vi "NavbalLabVIEW(15-5-21).vi"() -> ()   [LabVIEW 2010] (continued)
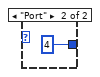
[diagram p2: hidden frame]
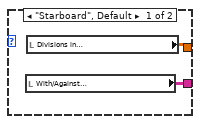
[diagram p4: hidden frame]
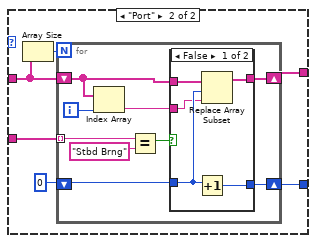
[diagram p6: hidden frame]
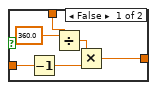
[diagram p10: hidden frame]
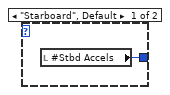
[diagram p11: hidden frame]
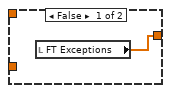
[diagram p12: hidden frame]
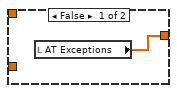
[diagram p13: hidden frame]
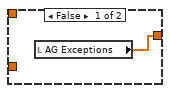
[diagram p14: hidden frame]
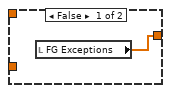
[diagram p15: hidden frame]
                  n2665 = Decrement(x=w3078) -> (x-1=w3116:dbl)
                  n2666 = Decrement(x=w3079) -> (x-1=w3115:dbl)
                  n2667 = Decrement(x=w3077) -> (x-1=w3117:dbl)
                  n2668 = Multiply(x=w3116, y=w3068) -> (x*y=w3090:dbl)
                  n2669 = Multiply(x=w3115, y=w3068) -> (x*y=w3080:dbl)
                  n2670 = Multiply(x=w3117, y=w3068) -> (x*y=w3109:dbl)
                  n2671 = Build Array (concatenate) "Percent"(w3137, w3138) -> (w3133:T3)
                  n2672 = Index Array(array=w3111, index (row)=w3080, index (col)=w3081) -> (element=w3112:bool)
                  n2673 = Index Array(array=w3111, index (row)=w3090, index (col)=w3091) -> (element=w3113:bool)
                  n2674 = Index Array(array=w3111, index (row)=w3109, index (col)=w3108) -> (element=w3114:bool)
                  n2675 = Index Array(array=w3076, index (row)=w3090, index (col)=w3091) -> (element=w3092:dbl)
                  n2676 = Index Array(array=w3076, index (row)=w3109, index (col)=w3108) -> (element=w3105:dbl)
                  n2677 = Index Array(array=w3076, index (row)=w3080, index (col)=w3081) -> (element=w3087:dbl)
                  n2678 = Greater Than 0?(x=w3092) -> (x > 0?=w3089:bool)
                  n2679 = Greater Than 0?(x=w3105) -> (x > 0?=w3106:bool)
                  n2680 = Greater Than 0?(x=w3087) -> (x > 0?=w3083:bool)
                  n2681 = Number To Fractional String(number=w3092, precision (6)=i16 1) -> (F-format string=w3093:string)  [unwired: 2 in]
                  n2682 = Number To Fractional String(number=w3105, precision (6)=i16 1) -> (F-format string=w3104:string)  [unwired: 2 in]
                  n2683 = Number To Fractional String(number=w3087, precision (6)=i16 1) -> (F-format string=w3086:string)  [unwired: 2 in]
                  n2684 = Concatenate Strings(w3093, " wt in hole") -> (w3088:string)
                  n2685 = Concatenate Strings(w3104, " wt in hole") -> (w3102:string)
                  n2686 = Concatenate Strings(w3086, " wt in hole") -> (w3082:string)
                  n2687 = Build Array (concatenate)(w3135, w3133) -> (w3134:T3)
                  n2688 = Select(t=w3082, s=w3083, f="  ") -> (s? t:f=w3096:string)
                  n2689 = Select(t=w3102, s=w3106, f="  ") -> (s? t:f=w3100:string)
                  n2690 = Select(t=w3088, s=w3089, f="  ") -> (s? t:f=w3098:string)
                  n2691 = Number To Fractional String(number=w3134, precision (6)=i16 3) -> (F-format string=w3132:string[][])  [unwired: 2 in]
                  n2692 = Build Array(w3129, w3129, w3129, w3129) -> (w3131:string[])
                  n2693 = Select(t=w3121, s=w3112, f=w3096) -> (s? t:f=w3124:string)
                  n2694 = Select(t=w3121, s=w3113, f=w3098) -> (s? t:f=w3123:string)
                  n2695 = Select(t=w3121, s=w3114, f=w3100) -> (s? t:f=w3122:string)
                  n2696 = Insert Into Array(array=w3132, index (row)=1, new element=w3131) -> (w3128:string[][])  [unwired: 1 in]
                  n2697 = Replace Array Subset(array=w3128, new element=w3129, index (row)=3 ("disabled index (row)"), index (col)=0 ("disabled index (col)")) -> (w3119:string[][])
                  n2698 = Build Array(w3124, "  ", w3123, w3122) -> (w3120:string[])
                  n2699 = Insert Into Array(array=w3119, index (col)=4 ("disabled index (col)"), new element=w3120) -> (w3118:string[][])  [unwired: 1 in]
                  n2700 = property on="Fwd Generator Balance Plane Split Options" class="MCListbox (strict)"("ItemNames"=w3118) -> ()  [unwired: 2 in, 2 out]
                  "FG Correction 1" <- w3069
                  "FG Correction 2A" <- w3072
                  "FG Correction 2B" <- w3071
                }
              }
            }
            "2wt-Exceptions" <- w2654
          }
        }
        n2701 = local read "AT Exceptions"() -> (w621:csg[])
        n2702 = local read "2wt-Exceptions"() -> (w620:csg[])
        n2703 = case shown="True" "Omit AT" {
          tunnel: w621 -> [_ w839]
          tunnel: w620 -> [_ w837]
          tunnel: [w833 w834] -> w619
          frame False {
            n2704 = local read "AT Exceptions"() -> (w833:csg[])
          }
          frame True {
            n2705 = Index Array(array=w837, index=0) -> (element=w835:csg)
            n2706 = Insert Into Array(array=w839, index=0, new element=w835) -> (w834:csg[])
          }
        }
        "AT Exceptions" <- w619
        n2707 = local read "FT Exceptions"() -> (w615:csg[])
        n2708 = local read "2wt-Exceptions"() -> (w616:csg[])
        n2709 = case shown="True" "Omit FT" {
          tunnel: w615 -> [_ w832]
          tunnel: w616 -> [_ w830]
          tunnel: [w826 w827] -> w617
          frame False {
            n2710 = local read "FT Exceptions"() -> (w826:csg[])
          }
          frame True {
            n2711 = Index Array(array=w830, index=1) -> (element=w828:csg)
            n2712 = Insert Into Array(array=w832, index=0, new element=w828) -> (w827:csg[])
          }
        }
        "FT Exceptions" <- w617
        n2713 = local read "AG Exceptions"() -> (w623:csg[])
        n2714 = local read "2wt-Exceptions"() -> (w624:csg[])
        n2715 = case shown="True" "Omit AG" {
          tunnel: w623 -> [_ w846]
          tunnel: w624 -> [_ w844]
          tunnel: [w840 w841] -> w625
          frame False {
            n2716 = local read "AG Exceptions"() -> (w840:csg[])
          }
          frame True {
            n2717 = Index Array(array=w844, index=2) -> (element=w842:csg)
            n2718 = Insert Into Array(array=w846, index=0, new element=w842) -> (w841:csg[])
          }
        }
        "AG Exceptions" <- w625
        n2719 = local read "FG Exceptions"() -> (w628:csg[])
        n2720 = local read "2wt-Exceptions"() -> (w627:csg[])
        n2721 = case shown="True" "Omit FG" {
          tunnel: w628 -> [_ w853]
          tunnel: w627 -> [_ w851]
          tunnel: [w847 w848] -> w626
          frame False {
            n2722 = local read "FG Exceptions"() -> (w847:csg[])
          }
          frame True {
            n2723 = Index Array(array=w851, index=3) -> (element=w849:csg)
            n2724 = Insert Into Array(array=w853, index=0, new element=w849) -> (w848:csg[])
          }
        }
        "FG Exceptions" <- w626
        n2725 = local read "Divisions in\nEach Plane"() -> (w636:T3)
        n2726 = local read "1st Available"() -> (w650:bool)
        n2727 = local read "2nd Available"() -> (w649:bool)
        n2728 = local read "3rd Available"() -> (w648:bool)
        n2729 = local read "4th Available"() -> (w647:bool)
        n2730 = case shown="True" w650 {
          tunnel: w636 -> [_ w1024]
          frame False {
          }
          frame True {
            n2731 = invoke on="Aft Turbine Balance Plane Split Options" class="MCListbox (strict)" method="Get DblClk Row"() -> ("Get Double-clicked Row"=w1025:i32)  [unwired: 3 in, 2 out]
            n2732 = Index Array(array=w1024, index (row)=0, index (col)=0 ("disabled index (col)")) -> (element=w1022:dbl)
            n2733 = case shown="2" w1025 {
              tunnel: w1022 -> [_ w1026 w1053]
              frame -2, Default {
                # "-2 is the variable value when no box is currently double clicked"
              }
              frame 0 {
                w1030 = 360.0 ("x")
                w1042 = 0 ("disabled index (col)")
                w1046 = 0 ("disabled index (col)")
                # "Update Pending weights Boolean Array\nwith selected split's locations"
                # "Update Inputs for Prediction tab\nto reflect selected weight split"
                # "Pull mass, Phase, and Location Data\nfrom listbox's array"
                # "Single Mass Option Selected"
                n2734 = local read "AT Correction 1"() -> (w1040:cdb)
                n2735 = Complex To Polar(r * e^(i*theta)=w1040) -> (r=w1039:dbl, theta=w1027:dbl)
                n2736 = Divide(x=w1027, y=3.141592653589793) -> (x/y=w1038:dbl)
                n2737 = local read "Correction Mag"() -> (w1047:T3)
                n2738 = Multiply ("Multiply.vi")(x=180.0, y=w1038) -> (x*y=w1033:dbl)
                n2739 = Add ("Add.vi")(x=w1033, y=w1030) -> (x+y=w1034:dbl)
                n2740 = Greater Than 0?(x=w1033) -> (x > 0?=w1035:bool)
                n2741 = Select(t=w1033, s=w1035, f=w1034) -> (s? t:f=w1032:dbl)
                n2742 = Divide(x=w1026, y=w1030) -> (x/y=w1031:dbl)
                n2743 = Replace Array Subset(array=w1047, new element=w1039, index (row)=w1046, index (col)=w1046) -> (w1045:T3)
                n2744 = Multiply ("Multiply.vi")(x=w1032, y=w1031) -> (x*y=w1029:dbl)
                n2745 = Increment(x=w1029) -> (x+1=w1028:dbl)
                n2746 = local read "Correction Loc"() -> (w1044:T3)
                n2747 = local write "Correction Mag"(w1045) -> ()
                n2748 = Replace Array Subset(array=w1044, new element=w1028, index (row)=w1042, index (col)=w1042) -> (w1043:T3)
                n2749 = local write "Correction Loc"(w1043) -> ()
                n2750 = property on="Aft Turbine Balance Plane Split Options" class="MCListbox (strict)"("SelColor"=u32 40727) -> ()  [unwired: 2 in, 2 out]
              }
              frame 2 {
                w1052 = 360.0 ("x")
                w1066 = 0 ("disabled index (col)")
                w1070 = 0 ("disabled index (col)")
                n2751 = local read "AT Correction 2A"() -> (w1048:cdb)
                n2752 = local read "AT Correction 2B"() -> (w1049:cdb)
                n2753 = local read "Correction Mag"() -> (w1071:T3)
                n2754 = Add ("Add.vi")(x=w1048, y=w1049) -> (x+y=w1065:cdb)
                n2755 = Complex To Polar ("Complex To Polar.vi")(r * e^(i*theta)=w1065) -> (r=w1064:dbl, theta=w1060:dbl)
                n2756 = Divide(x=w1060, y=3.141592653589793) -> (x/y=w1063:dbl)
                n2757 = Replace Array Subset(array=w1071, new element=w1064, index (row)=w1070, index (col)=w1070) -> (w1069:T3)
                n2758 = local write "Correction Mag"(w1069) -> ()
                n2759 = Multiply ("Multiply.vi")(x=180.0, y=w1063) -> (x*y=w1056:dbl)
                n2760 = local read "Correction Loc"() -> (w1068:T3)
                n2761 = Add ("Add.vi")(x=w1056, y=w1052) -> (x+y=w1057:dbl)
                n2762 = Greater Than 0?(x=w1056) -> (x > 0?=w1058:bool)
                n2763 = Select(t=w1056, s=w1058, f=w1057) -> (s? t:f=w1055:dbl)
                n2764 = Divide(x=w1053, y=w1052) -> (x/y=w1054:dbl)
                n2765 = Multiply ("Multiply.vi")(x=w1055, y=w1054) -> (x*y=w1051:dbl)
                n2766 = Increment(x=w1051) -> (x+1=w1050:dbl)
                n2767 = Replace Array Subset(array=w1068, new element=w1050, index (row)=w1066, index (col)=w1066) -> (w1067:T3)
                n2768 = local write "Correction Loc"(w1067) -> ()
                n2769 = property on="Aft Turbine Balance Plane Split Options" class="MCListbox (strict)"("SelColor"=u32 40727) -> ()  [unwired: 2 in, 2 out]
              }
            }
          }
        }
        n2770 = case shown="True" w649 {
          tunnel: w636 -> [_ w1073]
          frame False {
          }
          frame True {
            n2771 = invoke on="Fwd Turbine Balance Plane Split Options" class="MCListbox (strict)" method="Get DblClk Row"() -> ("Get Double-clicked Row"=w1076:i32)  [unwired: 3 in, 2 out]
            n2772 = Index Array(array=w1073, index (row)=1, index (col)=0 ("disabled index (col)")) -> (element=w1072:dbl)
            n2773 = case shown="0" w1076 {
              tunnel: w1072 -> [_ w1078 w1103]
              frame -2, Default {
              }
              frame 0 {
                w1084 = 360.0 ("x")
                n2774 = local read "FT Correction 1"() -> (w1082:cdb)
                n2775 = Complex To Polar(r * e^(i*theta)=w1082) -> (r=w1081:dbl, theta=w1077:dbl)
                n2776 = Divide(x=w1077, y=3.141592653589793) -> (x/y=w1092:dbl)
                n2777 = Multiply ("Multiply.vi")(x=180.0, y=w1092) -> (x*y=w1087:dbl)
                n2778 = Add ("Add.vi")(x=w1087, y=w1084) -> (x+y=w1088:dbl)
                n2779 = Divide(x=w1078, y=w1084) -> (x/y=w1085:dbl)
                n2780 = Greater Than 0?(x=w1087) -> (x > 0?=w1089:bool)
                n2781 = Select(t=w1087, s=w1089, f=w1088) -> (s? t:f=w1086:dbl)
                n2782 = local read "Correction Mag"() -> (w1100:T3)
                n2783 = local read "Correction Loc"() -> (w1097:T3)
                n2784 = Multiply ("Multiply.vi")(x=w1086, y=w1085) -> (x*y=w1083:dbl)
                n2785 = Increment(x=w1083) -> (x+1=w1079:dbl)
                n2786 = Replace Array Subset(array=w1097, new element=w1079, index (row)=1 ("disabled index (row)"), index (col)=0 ("disabled index (col)")) -> (w1096:T3)
                n2787 = Replace Array Subset(array=w1100, new element=w1081, index (row)=1 ("disabled index (row)"), index (col)=0 ("disabled index (col)")) -> (w1098:T3)
                n2788 = local write "Correction Loc"(w1096) -> ()
                n2789 = local write "Correction Mag"(w1098) -> ()
                n2790 = property on="Fwd Turbine Balance Plane Split Options" class="MCListbox (strict)"("SelColor"=u32 40727) -> ()  [unwired: 2 in, 2 out]
              }
              frame 2 {
                w1106 = 360.0 ("x")
                n2791 = local read "FT Correction 2A"() -> (w1102:cdb)
                n2792 = local read "FT Correction 2B"() -> (w1101:cdb)
                n2793 = Add(x=w1102, y=w1101) -> (x+y=w1120:cdb)
                n2794 = Complex To Polar(r * e^(i*theta)=w1120) -> (r=w1119:dbl, theta=w1115:dbl)
                n2795 = local read "Correction Mag"() -> (w1126:T3)
                n2796 = Divide(x=w1115, y=3.141592653589793) -> (x/y=w1118:dbl)
                n2797 = Multiply ("Multiply.vi")(x=180.0, y=w1118) -> (x*y=w1109:dbl)
                n2798 = local read "Correction Loc"() -> (w1123:T3)
                n2799 = Add(x=w1109, y=w1106) -> (x+y=w1110:dbl)
                n2800 = Replace Array Subset(array=w1126, new element=w1119, index (row)=1 ("disabled index (row)"), index (col)=0 ("disabled index (col)")) -> (w1124:T3)
                n2801 = Greater Than 0?(x=w1109) -> (x > 0?=w1111:bool)
                n2802 = local write "Correction Mag"(w1124) -> ()
                n2803 = Select(t=w1109, s=w1111, f=w1110) -> (s? t:f=w1105:dbl)
                n2804 = Divide(x=w1103, y=w1106) -> (x/y=w1107:dbl)
                n2805 = Multiply ("Multiply.vi")(x=w1105, y=w1107) -> (x*y=w1108:dbl)
                n2806 = Increment(x=w1108) -> (x+1=w1104:dbl)
                n2807 = Replace Array Subset(array=w1123, new element=w1104, index (row)=1 ("disabled index (row)"), index (col)=0 ("disabled index (col)")) -> (w1122:T3)
                n2808 = local write "Correction Loc"(w1122) -> ()
                n2809 = property on="Fwd Turbine Balance Plane Split Options" class="MCListbox (strict)"("SelColor"=u32 40727) -> ()  [unwired: 2 in, 2 out]
              }
            }
          }
        }
        n2810 = case shown="True" w648 {
          tunnel: w636 -> [_ w1128]
          frame False {
          }
          frame True {
            n2811 = invoke on="Aft Generator Balance Plane Split Options" class="MCListbox (strict)" method="Get DblClk Row"() -> ("Get Double-clicked Row"=w1131:i32)  [unwired: 3 in, 2 out]
            n2812 = Index Array(array=w1128, index (row)=2, index (col)=0 ("disabled index (col)")) -> (element=w1127:dbl)
            n2813 = case shown="2" w1131 {
              tunnel: w1127 -> [_ w1133 w1157]
              frame -2, Default {
              }
              frame 0 {
                w1143 = 360.0 ("x")
                n2814 = local read "AG Correction 1"() -> (w1146:cdb)
                n2815 = Complex To Polar(r * e^(i*theta)=w1146) -> (r=w1145:dbl, theta=w1134:dbl)
                n2816 = Divide(x=w1134, y=3.141592653589793) -> (x/y=w1135:dbl)
                n2817 = Multiply ("Multiply.vi")(x=180.0, y=w1135) -> (x*y=w1140:dbl)
                n2818 = Greater Than 0?(x=w1140) -> (x > 0?=w1138:bool)
                n2819 = local read "Correction Mag"() -> (w1155:T3)
                n2820 = Add ("Add.vi")(x=w1140, y=w1143) -> (x+y=w1139:dbl)
                n2821 = Select(t=w1140, s=w1138, f=w1139) -> (s? t:f=w1141:dbl)
                n2822 = Divide(x=w1133, y=w1143) -> (x/y=w1142:dbl)
                n2823 = Multiply ("Multiply.vi")(x=w1141, y=w1142) -> (x*y=w1144:dbl)
                n2824 = Increment(x=w1144) -> (x+1=w1132:dbl)
                n2825 = Replace Array Subset(array=w1155, new element=w1145, index (row)=2 ("disabled index (row)"), index (col)=0 ("disabled index (col)")) -> (w1153:T3)
                n2826 = local read "Correction Loc"() -> (w1152:T3)
                n2827 = local write "Correction Mag"(w1153) -> ()
                n2828 = Replace Array Subset(array=w1152, new element=w1132, index (row)=2 ("disabled index (row)"), index (col)=0 ("disabled index (col)")) -> (w1151:T3)
                n2829 = local write "Correction Loc"(w1151) -> ()
                n2830 = property on="Aft Generator Balance Plane Split Options" class="MCListbox (strict)"("SelColor"=u32 40727) -> ()  [unwired: 2 in, 2 out]
              }
              frame 2 {
                w1156 = 360.0 ("x")
                n2831 = local read "AG Correction 2A"() -> (w1159:cdb)
                n2832 = local read "AG Correction 2B"() -> (w1158:cdb)
                n2833 = Add(x=w1159, y=w1158) -> (x+y=w1175:cdb)
                n2834 = Complex To Polar(r * e^(i*theta)=w1175) -> (r=w1174:dbl, theta=w1170:dbl)
                n2835 = local read "Correction Mag"() -> (w1181:T3)
                n2836 = Divide(x=w1170, y=3.141592653589793) -> (x/y=w1173:dbl)
                n2837 = Multiply ("Multiply.vi")(x=180.0, y=w1173) -> (x*y=w1164:dbl)
                n2838 = Add(x=w1164, y=w1156) -> (x+y=w1165:dbl)
                n2839 = Greater Than 0?(x=w1164) -> (x > 0?=w1166:bool)
                n2840 = local read "Correction Loc"() -> (w1178:T3)
                n2841 = Select(t=w1164, s=w1166, f=w1165) -> (s? t:f=w1161:dbl)
                n2842 = Replace Array Subset(array=w1181, new element=w1174, index (row)=2 ("disabled index (row)"), index (col)=0 ("disabled index (col)")) -> (w1179:T3)
                n2843 = Divide(x=w1157, y=w1156) -> (x/y=w1163:dbl)
                n2844 = local write "Correction Mag"(w1179) -> ()
                n2845 = Multiply ("Multiply.vi")(x=w1161, y=w1163) -> (x*y=w1162:dbl)
                n2846 = Increment(x=w1162) -> (x+1=w1160:dbl)
                n2847 = Replace Array Subset(array=w1178, new element=w1160, index (row)=2 ("disabled index (row)"), index (col)=0 ("disabled index (col)")) -> (w1177:T3)
                n2848 = local write "Correction Loc"(w1177) -> ()
                n2849 = property on="Aft Generator Balance Plane Split Options" class="MCListbox (strict)"("SelColor"=u32 40727) -> ()  [unwired: 2 in, 2 out]
              }
            }
          }
        }
        n2850 = case shown="True" w647 {
          tunnel: w636 -> [_ w1183]
          frame False {
          }
          frame True {
            n2851 = invoke on="Fwd Generator Balance Plane Split Options" class="MCListbox (strict)" method="Get DblClk Row"() -> ("Get Double-clicked Row"=w1186:i32)  [unwired: 3 in, 2 out]
            n2852 = Index Array(array=w1183, index (row)=2, index (col)=0 ("disabled index (col)")) -> (element=w1182:dbl)
            n2853 = case shown="2" w1186 {
              tunnel: w1182 -> [_ w1191 w1212]
              frame -2, Default {
              }
              frame 0 {
                w1193 = 360.0 ("x")
                n2854 = local read "FG Correction 1"() -> (w1190:cdb)
                n2855 = Complex To Polar(r * e^(i*theta)=w1190) -> (r=w1189:dbl, theta=w1188:dbl)
                n2856 = Divide(x=w1188, y=3.141592653589793) -> (x/y=w1201:dbl)
                n2857 = Multiply ("Multiply.vi")(x=180.0, y=w1201) -> (x*y=w1196:dbl)
                n2858 = local read "Correction Mag"() -> (w1210:T3)
                n2859 = Add ("Add.vi")(x=w1196, y=w1193) -> (x+y=w1197:dbl)
                n2860 = Greater Than 0?(x=w1196) -> (x > 0?=w1198:bool)
                n2861 = Select(t=w1196, s=w1198, f=w1197) -> (s? t:f=w1195:dbl)
                n2862 = Divide(x=w1191, y=w1193) -> (x/y=w1194:dbl)
                n2863 = Multiply ("Multiply.vi")(x=w1195, y=w1194) -> (x*y=w1192:dbl)
                n2864 = Increment(x=w1192) -> (x+1=w1187:dbl)
                n2865 = Replace Array Subset(array=w1210, new element=w1189, index (row)=3 ("disabled index (row)"), index (col)=0 ("disabled index (col)")) -> (w1208:T3)
                n2866 = local read "Correction Loc"() -> (w1207:T3)
                n2867 = local write "Correction Mag"(w1208) -> ()
                n2868 = Replace Array Subset(array=w1207, new element=w1187, index (row)=3 ("disabled index (row)"), index (col)=0 ("disabled index (col)")) -> (w1206:T3)
                n2869 = local write "Correction Loc"(w1206) -> ()
                n2870 = property on="Fwd Generator Balance Plane Split Options" class="MCListbox (strict)"("SelColor"=u32 40727) -> ()  [unwired: 2 in, 2 out]
              }
              frame 2 {
                w1215 = 360.0 ("x")
                n2871 = local read "FG Correction 2A"() -> (w1225:cdb)
                n2872 = local read "FG Correction 2B"() -> (w1224:cdb)
                n2873 = Add(x=w1225, y=w1224) -> (x+y=w1230:cdb)
                n2874 = Complex To Polar(r * e^(i*theta)=w1230) -> (r=w1229:dbl, theta=w1213:dbl)
                n2875 = local read "Correction Mag"() -> (w1236:T3)
                n2876 = Divide(x=w1213, y=3.141592653589793) -> (x/y=w1223:dbl)
                n2877 = Multiply ("Multiply.vi")(x=180.0, y=w1223) -> (x*y=w1218:dbl)
                n2878 = Greater Than 0?(x=w1218) -> (x > 0?=w1220:bool)
                n2879 = Add ("Add.vi")(x=w1218, y=w1215) -> (x+y=w1219:dbl)
                n2880 = Divide(x=w1212, y=w1215) -> (x/y=w1216:dbl)
                n2881 = Select(t=w1218, s=w1220, f=w1219) -> (s? t:f=w1217:dbl)
                n2882 = Replace Array Subset(array=w1236, new element=w1229, index (row)=3 ("disabled index (row)"), index (col)=0 ("disabled index (col)")) -> (w1234:T3)
                n2883 = local read "Correction Loc"() -> (w1233:T3)
                n2884 = Multiply ("Multiply.vi")(x=w1217, y=w1216) -> (x*y=w1214:dbl)
                n2885 = local write "Correction Mag"(w1234) -> ()
                n2886 = Increment(x=w1214) -> (x+1=w1211:dbl)
                n2887 = Replace Array Subset(array=w1233, new element=w1211, index (row)=3 ("disabled index (row)"), index (col)=0 ("disabled index (col)")) -> (w1232:T3)
                n2888 = property on="Fwd Generator Balance Plane Split Options" class="MCListbox (strict)"("SelColor"=u32 40727) -> ()  [unwired: 2 in, 2 out]
                n2889 = local write "Correction Loc"(w1232) -> ()
              }
            }
          }
        }
      }
    }
    n2890 = case "Refresh Run Name Listbox on Import Mag-Phase Tab" shown="True" w348 {
      tunnel: w363 -> [_ w461]
      tunnel: w359 -> [_ w460]
      tunnel: "Select Side to Analyze" -> [_ w379]
      frame False {
      }
      frame True {
        w404 = sgl[] []  # Empty Array
        w409 = sgl[] []  # Empty Array
        w414 = sgl[] []  # Empty Array
        w421 = sgl[] []  # Empty Array
        w458 = sgl[] []  # Empty Array
        # "2. Use every other\ncolumn"
        # "1. Choose first\nthree rows"
        n2891 = call <vilib>:"New Report.vi"("report type"=T11."Excel", "template (empty)"=w461) -> ("report out"=w434:refnum<class "NI_report.lvclass">, "error out"=w433:errorcluster)  [unwired: 12 in]
        n2892 = call <vilib>:"Excel Get Worksheet.vi"("report in"=w434, "worksheet index (0)"=w460, "error in (no error)"=w433) -> ("report out"=w536:refnum<class "NI_report.lvclass">, "error out"=w535:errorcluster)  [unwired: 11 out]
        n2893 = call <vilib>:"Excel Get Worksheet.vi"("report in"=w434, "worksheet index (0)"=1, "error in (no error)"=w433) -> ("report out"=w512:refnum<class "NI_report.lvclass">, "error out"=w511:errorcluster)  [unwired: 11 out]
        n2894 = local read "Weight Category FT"() -> (w495:u16)
        n2895 = call <vilib>:"Excel Get Worksheet.vi"("report in"=w434, "worksheet index (0)"=1, "error in (no error)"=w433) -> ("report out"=w456:refnum<class "NI_report.lvclass">, "error out"=w457:errorcluster)  [unwired: 11 out]
        n2896 = call-poly <vilib>:"Excel Get Data.vi"("report in"=w512, "data type"=string[][] [], "start (-1, -1)"=cluster{"row":i32, "column":i32} {"row"=0, "column"=0}, "end (-1, -1)"=cluster{"row":i32, "column":i32} {"row"=0, "column"=15} ("start (-1, -1)"), "error in (no error)"=w511) -> ("data"=w507:string[][])  [unwired: 10 out]
        n2897 = call <vilib>:"Excel Get Last Row.vi"("report in"=w456, "error in (no error)"=w457) -> ("report out"=w454:refnum<class "NI_report.lvclass">, "MS Office parameters out"=w455:T14, "error out"=w453:errorcluster)  [unwired: 11 in]
        n2898 = Increment(x="No. Runs") -> (x+1=w500:i32)
        n2899 = Multiply(x=w500, y=2) -> (x*y=w502:i32)
        n2900 = Index Array(array=w507, index (row)=0) -> (element=w505:string[])  [unwired: 1 in]
        n2901 = Unbundle(w455) -> ("position (Excel)"=w493:cluster{"row":i32, "column":i32})  [unwired: 2 out]
        n2902 = Bundle("row"=2, w502) -> (w501:cluster{"row":i32, i32})  [unwired: 1 in]
        n2903 = call-poly <vilib>:"Excel Get Data.vi"("report in"=w536, "data type"=string[][] [], "start (-1, -1)"=cluster{"row":i32, "column":i32} {"row"=0, "column"=1}, "end (-1, -1)"=w501, "error in (no error)"=w535) -> ("data"=w514:string[][])  [unwired: 10 out]
        n2904 = Transpose 2D Array(2D array=w514) -> (transposed array=w531:string[][])
        n2905 = Unbundle(w493) -> ("row"=w494:i32)  [unwired: 1 out]
        n2906 = Bundle(1, "Weight Category FT"=w495) -> (w492:cluster{i32, "Weight Category FT":u16})  [unwired: 1 in]
        n2907 = property on="Weight Category AT" class="Ring (strict)"("Strings []"=w505) -> ()  [unwired: 2 in, 2 out]
        n2908 = Bundle("row"=w494, "Weight Category FT"=w495) -> (w496:cluster{"row":i32, "Weight Category FT":u16})  [unwired: 1 in]
        n2909 = call-poly <vilib>:"Excel Get Data.vi"("report in"=w454, "data type"=sgl[][] [], "start (-1, -1)"=w492, "end (-1, -1)"=w496, "error in (no error)"=w453) -> ("data"=w498:dbl[][])  [unwired: 10 out]
        n2910 = Index Array(array=w498, index (col)=0 ("disabled index (col)")) -> (element=w416:dbl[])  [unwired: 1 in]
        n2911 = for {
          shift-right: [w554] -> w420
          shift-left: w421 -> [w555]
          tunnel: w416 -> [w553] mode=indexing
          n2912 = Build Array (concatenate)(w555, w553) -> (w554:dbl[])
        }
        n2913 = Insert Into Array(array=w420, index=0, new element=0 ("new element/subarray")) -> (w417:dbl[])
        n2914 = Index Array(array=w531, index (col)=1 ("disabled index (col)")) -> (element=w530:string[])  [unwired: 1 in]
        n2915 = Index Array(array=w531, index (col)=2 ("disabled index (col)")) -> (element=w529:string[])  [unwired: 1 in]
        n2916 = Index Array(array=w531, index (col)=0 ("disabled index (col)")) -> (element=w516:string[])  [unwired: 1 in]
        n2917 = Sort 1D Array(array=w417) -> (sorted array=→"FT Weights":dbl[])
        n2918 = Decimate 1D Array(w516) -> (w513:string[])  [unwired: 1 out]
        n2919 = Decimate 1D Array(w529) -> (w524:string[])  [unwired: 1 out]
        n2920 = Decimate 1D Array(w530) -> (w526:string[])  [unwired: 1 out]
        n2921 = Array Size(array=w513) -> (size(s)=w515:i32)
        n2922 = property on="Weight Category FT" class="Ring (strict)"("Strings []"=w505) -> ()  [unwired: 2 in, 2 out]
        n2923 = Reshape Array(w524, w515, 1 ("dimension size")) -> (w518:string[][])
        n2924 = Reshape Array(w513, w515, 1 ("dimension size")) -> (w523:string[][])
        n2925 = Reshape Array(w526, w515, 1 ("dimension size")) -> (w521:string[][])
        n2926 = property on="Start Point:" class="Ring (strict)"("Strings []"=w513) -> ()  [unwired: 2 in, 2 out]
        n2927 = Insert Into Array(array=w523, index (col)=1 ("disabled index (col)"), new element=w521) -> (w519:string[][])  [unwired: 1 in]
        n2928 = local read "Weight Category AG"() -> (w485:u16)
        n2929 = property on="Weight Category AG" class="Ring (strict)"("Strings []"=w505) -> ()  [unwired: 2 in, 2 out]
        n2930 = Insert Into Array(array=w519, index (col)=2 ("disabled index (col)"), new element=w518) -> (w517:string[][])  [unwired: 1 in]
        n2931 = property on="Multicolumn Listbox" class="MCListbox (strict)"("ItemNames"=w517) -> ()  [unwired: 2 in, 2 out]
        n2932 = Unbundle(w455) -> ("position (Excel)"=w483:cluster{"row":i32, "column":i32})  [unwired: 2 out]
        n2933 = property on="Weight Category FG" class="Ring (strict)"("Strings []"=w505) -> ()  [unwired: 2 in, 2 out]
        n2934 = Unbundle(w483) -> ("row"=w484:i32)  [unwired: 1 out]
        n2935 = Bundle(1, "Weight Category AG"=w485) -> (w482:cluster{i32, "Weight Category AG":u16})  [unwired: 1 in]
        n2936 = Bundle("row"=w484, "Weight Category AG"=w485) -> (w486:cluster{"row":i32, "Weight Category AG":u16})  [unwired: 1 in]
        n2937 = call-poly <vilib>:"Excel Get Data.vi"("report in"=w454, "data type"=sgl[][] [], "start (-1, -1)"=w482, "end (-1, -1)"=w486, "error in (no error)"=w453) -> ("data"=w488:dbl[][])  [unwired: 10 out]
        n2938 = Index Array(array=w488, index (col)=0 ("disabled index (col)")) -> (element=w396:dbl[])  [unwired: 1 in]
        n2939 = for {
          shift-right: [w551] -> w411
          shift-left: w414 -> [w552]
          tunnel: w396 -> [w550] mode=indexing
          n2940 = Build Array (concatenate)(w552, w550) -> (w551:dbl[])
        }
        n2941 = Insert Into Array(array=w411, index=0, new element=0 ("new element/subarray")) -> (w410:dbl[])
        n2942 = Sort 1D Array(array=w410) -> (sorted array=→"AG Weights":dbl[])
        n2943 = local write "AT Exceptions"(w458) -> ()
        n2944 = local write "FT Exceptions"(w458) -> ()
        n2945 = local write "AG Exceptions"(w458) -> ()
        n2946 = local write "FG Exceptions"(w458) -> ()
        n2947 = local read "Weight Category FG"() -> (w476:u16)
        n2948 = case shown="\"Port\"" w379 {
          tunnel: [w541 w543] -> w378
          tunnel: [w540 w542] -> w377
          frame "Starboard", Default {
            n2949 = local read "With/Against\nRotation S"() -> (w540:string[][])
            n2950 = local read "Divisions in\nEach Plane S"() -> (w541:T3)
          }
          frame "Port" {
            n2951 = local read "Divisions in\nEach Plane P"() -> (w543:T3)
            n2952 = local read "With/Against\nRotation P"() -> (w542:string[][])
          }
        }
        n2953 = Unbundle(w455) -> ("position (Excel)"=w474:cluster{"row":i32, "column":i32})  [unwired: 2 out]
        n2954 = local write "Divisions in\nEach Plane"(w378) -> ()
        n2955 = local write "With/Against\nRotation"(w377) -> ()
        n2956 = Unbundle(w474) -> ("row"=w475:i32)  [unwired: 1 out]
        n2957 = Bundle(1, "Weight Category FG"=w476) -> (w473:cluster{i32, "Weight Category FG":u16})  [unwired: 1 in]
        n2958 = Bundle("row"=w475, "Weight Category FG"=w476) -> (w477:cluster{"row":i32, "Weight Category FG":u16})  [unwired: 1 in]
        n2959 = call-poly <vilib>:"Excel Get Data.vi"("report in"=w454, "data type"=sgl[][] [], "start (-1, -1)"=w473, "end (-1, -1)"=w477, "error in (no error)"=w453) -> ("data"=w478:dbl[][])  [unwired: 10 out]
        n2960 = Index Array(array=w478, index (col)=0 ("disabled index (col)")) -> (element=w398:dbl[])  [unwired: 1 in]
        n2961 = for {
          shift-right: [w548] -> w406
          shift-left: w409 -> [w549]
          tunnel: w398 -> [w547] mode=indexing
          n2962 = Build Array (concatenate)(w549, w547) -> (w548:dbl[])
        }
        n2963 = Insert Into Array(array=w406, index=0, new element=0 ("new element/subarray")) -> (w405:dbl[])
        n2964 = Sort 1D Array(array=w405) -> (sorted array=→"FG Weights":dbl[])
        n2965 = local read "Sensor Info"() -> (w426:string[][])
        n2966 = local read "Weight Category AT"() -> (w467:u16)
        n2967 = Index Array(array=w426, index (col)=0 ("disabled index (col)")) -> (element=w429:string[])  [unwired: 1 in]
        n2968 = Index Array(array=w426, index (col)=2 ("disabled index (col)")) -> (element=w425:string[])  [unwired: 1 in]
        n2969 = case shown="\"Starboard\", Default" w379 {
          tunnel: w429 -> [w560 w582]
          tunnel: [w558 w580] -> w424
          tunnel: w425 -> [w559 w581]
          tunnel: [w556 w578] -> w423
          frame "Starboard", Default {
            n2970 = Array Size(array=w560) -> (size(s)=w561:i32)
            n2971 = for {
              N: w561 -> [_]
              tunnel: w559 -> [w570] mode=indexing
              shift-right: [w567] -> w558
              shift-left: w560 -> [w564]
              shift-right: [w565] -> w556
              shift-left: 0 -> [w566]
              i -> [w563]
              n2972 = Index Array(array=w564, index=w563) -> (element=w562:string)
              n2973 = Equal?(x=w570, y="Port Brng") -> (x = y?=w568:bool)
              n2974 = case shown="False" w568 {
                tunnel: [w574 w577] -> w567
                tunnel: w564 -> [w575 w577]
                tunnel: w566 -> [w572 w576]
                tunnel: [w573 w576] -> w565
                tunnel: w562 -> [w571 _]
                frame False {
                  n2975 = Increment(x=w572) -> (x+1=w573:i32)
                  n2976 = Replace Array Subset(array=w575, new element=w571, index=w572) -> (w574:string[])
                }
                frame True {
                }
              }
            }
          }
          frame "Port" {
            n2977 = Array Size(array=w582) -> (size(s)=w583:i32)
            n2978 = for {
              N: w583 -> [_]
              tunnel: w581 -> [w592] mode=indexing
              shift-right: [w589] -> w580
              shift-left: w582 -> [w586]
              shift-right: [w587] -> w578
              shift-left: 0 -> [w588]
              i -> [w585]
              n2979 = Index Array(array=w586, index=w585) -> (element=w584:string)
              n2980 = Equal?(x=w592, y="Stbd Brng") -> (x = y?=w590:bool)
              n2981 = case shown="False" w590 {
                tunnel: [w596 w599] -> w589
                tunnel: w586 -> [w597 w599]
                tunnel: w588 -> [w594 w598]
                tunnel: [w595 w598] -> w587
                tunnel: w584 -> [w593 _]
                frame False {
                  n2982 = Increment(x=w594) -> (x+1=w595:i32)
                  n2983 = Replace Array Subset(array=w597, new element=w593, index=w594) -> (w596:string[])
                }
                frame True {
                }
              }
            }
          }
        }
        n2984 = Unbundle(w455) -> ("position (Excel)"=w465:cluster{"row":i32, "column":i32})  [unwired: 2 out]
        n2985 = Unbundle(w465) -> ("row"=w466:i32)  [unwired: 1 out]
        n2986 = Bundle(1, "Weight Category AT"=w467) -> (w464:cluster{i32, "Weight Category AT":u16})  [unwired: 1 in]
        n2987 = Bundle("row"=w466, "Weight Category AT"=w467) -> (w468:cluster{"row":i32, "Weight Category AT":u16})  [unwired: 1 in]
        n2988 = call-poly <vilib>:"Excel Get Data.vi"("report in"=w454, "data type"=sgl[][] [], "start (-1, -1)"=w464, "end (-1, -1)"=w468, "error in (no error)"=w453) -> ("data"=w470:dbl[][])  [unwired: 10 out]
        n2989 = Index Array(array=w470, index (col)=0 ("disabled index (col)")) -> (element=w395:dbl[])  [unwired: 1 in]
        n2990 = for {
          shift-right: [w545] -> w401
          shift-left: w404 -> [w546]
          tunnel: w395 -> [w544] mode=indexing
          n2991 = Build Array (concatenate)(w546, w544) -> (w545:dbl[])
        }
        n2992 = Insert Into Array(array=w401, index=0, new element=0 ("new element/subarray")) -> (w400:dbl[])
        n2993 = Sort 1D Array(array=w400) -> (sorted array=→"AT Weights":dbl[])
        n2994 = Reshape Array(w424, w423) -> (→"Sensor Column":string[])
        n2995 = call <vilib>:"Excel Get Worksheet.vi"("report in"=w434, "worksheet index (0)"=2, "error in (no error)"=w433) -> ("report out"=w382:refnum<class "NI_report.lvclass">, "error out"=w381:errorcluster)  [unwired: 11 out]
        n2996 = call <vilib>:"Excel Get Last Row.vi"("report in"=w382, "error in (no error)"=w381) -> ("report out"=w451:refnum<class "NI_report.lvclass">, "MS Office parameters out"=w448:T14, "error out"=w450:errorcluster)  [unwired: 11 in]
        n2997 = Unbundle(w448) -> ("position (Excel)"=w449:cluster{"row":i32, "column":i32})  [unwired: 2 out]
        n2998 = call-poly <vilib>:"Excel Get Data.vi"("report in"=w382, "data type"=sgl[][] [], "start (-1, -1)"=cluster{"start row":i32, "start column":i32} {"start row"=3, "start column"=0} ("start (0, 0)"), "end (-1, -1)"=cluster{"start row":i32, "start column":i32} {"start row"=4, "start column"=0} ("start (0, 0)"), "error in (no error)"=w381) -> ("data"=w386:dbl[][])  [unwired: 10 out]
        n2999 = Unbundle(w449) -> ("row"=w439:i32)  [unwired: 1 out]
        n3000 = Index Array(array=w386, index (row)=1, index (col)=0) -> (element=w385:dbl)
        n3001 = Index Array(array=w386, index (row)=0, index (col)=0) -> (element=w384:dbl)
        n3002 = Subtract(x=w439, y=2.0) -> (x-y=w431:dbl)
        n3003 = Bundle("row"=w439, "start column"=8) -> (w444:cluster{"row":i32, "start column":i32})  [unwired: 1 in]
        n3004 = call-poly <vilib>:"Excel Get Data.vi"("report in"=w451, "data type"=sgl[][] [], "start (-1, -1)"=cluster{"start row":i32, "start column":i32} {"start row"=3, "start column"=1} ("start (0, 0)"), "end (-1, -1)"=w444, "error in (no error)"=w450) -> ("data"=w435:dbl[][])  [unwired: 10 out]
        n3005 = Subtract(x=w385, y=w384) -> (x-y=w383:dbl)
        n3006 = Reciprocal(x=w383) -> (1/x=w380:dbl)
        n3007 = Array Subset(array=w435, index (row)=0 ("index"), length (row)=w431, index (col)=0 ("index"), length (col)=4 ("length")) -> (w442:dbl[][])
        n3008 = Array Subset(array=w435, index (row)=0 ("index"), length (row)=w431, index (col)=4 ("index"), length (col)=4 ("length")) -> (w436:dbl[][])
        n3009 = property on="Holes/Division" class="DigNum (strict)"("Value"=w380) -> ()  [unwired: 2 in, 2 out]
        n3010 = local write "Existing Plane Wts Port"(w442) -> ()
        n3011 = local write "Existing Plane Wts Stbd"(w436) -> ()
        "DataTab" <- w460
      }
    }
  }
